vi "Segment.vi"(5 "仪器地址":u32, 7 "File ID":string, 9 "Segment 1 to 99":T2(array[cluster]), 11 "Segment 0":T1) -> (3 "Array":string[](array[string]))   [LabVIEW 2010, in "DCP551.lvlib"]
uses:
  DCP551.lvlib
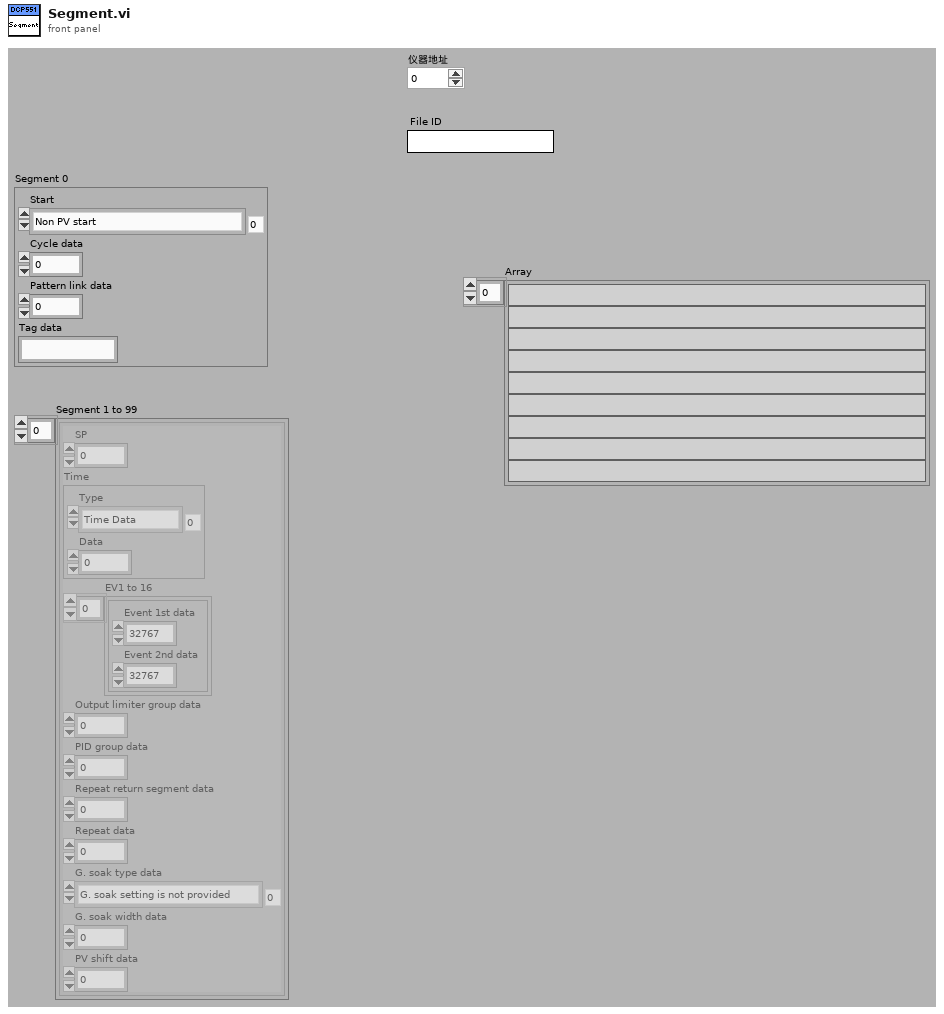
[diagram p1: front panel]
types:
  T1 = cluster{"Start":enum16{"Non PV start", "Upward PV tart", "Downward PV start", "Either upward of downward PV start"}, "Cycle data":i32, "Pattern link data":i32, "Tag data":string}
  T2 = cluster{"SP":dbl, "Time":cluster{"Type":enum16{"Time Data", "delta Dtada", "SP Data"}, "Data":i32}, "EV1 to 16":cluster{"Event 1st data":i32, "Event 2nd data":i32}[], "Output limiter group data":i32, "PID group data":i32, "Repeat return segment data":i32, "Repeat data":i32, "G. soak type data":enum16{"G. soak setting is not provided", "Segment start point", "Segment end point", "Total segment"}, "G. soak width data":i32, "PV shift data":i32}[]
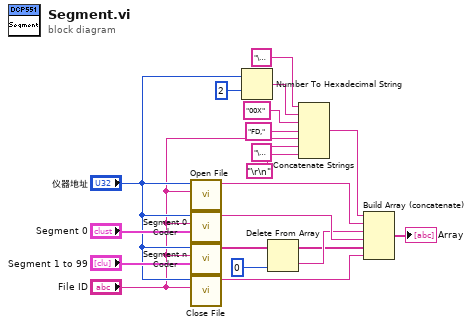
[diagram p0: block diagram]
diagram:
  n1 = call "Open File.vi"("File ID"="File ID", "仪器地址"="仪器地址") -> ("OutPut"=w19:string)  [unwired: 9 in]
  n2 = call "Segment 0 Coder.vi"("Segment 0"="Segment 0", "File ID"="File ID", "仪器地址"="仪器地址") -> ("Output"=w13:string)  [unwired: 8 in]
  n3 = call "Segment n Coder.vi"("Segment 1 to 99"="Segment 1 to 99", "File ID"="File ID", "仪器地址"="仪器地址") -> ("Output"=w15:string[])  [unwired: 8 in]
  n4 = call "Close File.vi"("File ID"="File ID", "仪器地址"="仪器地址") -> ("Output"=w18:string)  [unwired: 9 in]
  n5 = Number To Hexadecimal String(1:i16 2 ("width (-)"), 2:"仪器地址") -> (0:w8:string)
  n6 = Delete From Array(array=w15, index=0) -> (deleted portion=w12:string, array with subset deleted=w11:string[])  [unwired: 1 in]
  n7 = Concatenate Strings("\u0002" ("string"), w8, "00X" ("string"), "FD," ("string"), "File ID", "\u0003" ("string"), "\r\n") -> (w1:string)
  n8 = Build Array (concatenate)(w1, w19, w12, w13, w11, w18) -> (→"Array":string[])
